vi "bson_alloc.vi"() -> (3 "bson_iterator ptr":u32)   [LabVIEW 2013]
uses:
  mongo-c-driver/libmongoc.so
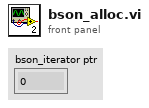
[diagram p1: front panel]
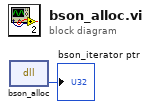
[diagram p0: block diagram]
diagram:
  n1 = dll-call lib="home/scot/dev/git/mongo-c-driver/libmongoc.so" fn="bson_alloc"() -> ("bson ptr"=→"bson_iterator ptr":u32)  [unwired: 3 in, 2 out]
